vi "Diagnostic.vi"() -> ()   [LabVIEW 2018]
uses:
  Type/_GUI Method.ctl
  Type/_Lens Property.ctl
  Type/_Mass Range Property.ctl
  Type/_Mass Range Parameters.ctl
  Type/_RT Res Type.ctl
  Type/_Run Mode.ctl
  Type/_Run State.ctl
  Type/_File Type.ctl
  Type/_RT Command.ctl
  Type/_Data Operation.ctl
  Type/_Run Module.ctl
  Configuration/_Global Configuration.vi
  <vilib>/Utility/config.llb/Read Key (Path).vi
  <vilib>/Utility/config.llb/Read Key (String).vi
  <vilib>/printing/ReportDocExtensions.llb/Append Front Panel Image to Report (path).vi
  <vilib>/Utility/config.llb/Write Key (Path).vi
  <vilib>/Utility/config.llb/Write Key (String).vi
  <vilib>/Utility/miscctls.llb/LVRectTypeDef.ctl
  <vilib>/Utility/NIReport.llb/NI_report.lvclass
  <vilib>/Utility/NIReport.llb/NI_ReportGenerationCore.lvlib
  <vilib>/Utility/config.llb/NI_LVConfig.lvlib
panel:
  out "Error Out":errorcluster
  in  "Run Mode":T1
  in  "Q2DC EN":bool
  in  "Count1":dbl=400.0 caption="Lens Value" format="%#.3f"
  in  "Count2":dbl=400.0 caption="High Value" format="%#.3f"
  in  "Time1":dbl=1.0 caption="Low Dwell (ms)" format="%#.3f"
  in  "Time2":dbl=1.0 caption="High Dwell (ms)" format="%#.3f"
  in  "Scans":i32=1
  in  "Step Size":dbl=-1.0 format="%#.3f"
  in  "Scan Type":u8(ring) items=["Single", "Dual", "Ramp"]
  in  "Unit":bool
  in  "Q1DC EN":bool
  in  "Q1 POL":bool
  in  "Q2 POL":bool
  out "DAC Value":i32=98187
  in  "Lens Table":i32(listbox)
  in  "Swtich Polarity":bool
  in  "Run":bool
  out "Dual Run":bool
  out "Spectrum":cluster{"Mass":dbl[], "Data in cps":dbl[]}[](graph)=[{"Mass"=[664.0], "Data in cps"=[]}, {"Mass"=[800.0], "Data in cps"=[]}, {"Mass"=[700.0], "Data in cps"=[]}]
  in  "Cancel":bool
  in  "NewMethod":bool
  in  "Method Path":path
  in  "Method":T2={"Lenses"=[{"Scan Type"=0, "Scans"=1, "Time 1"=1.0, "Time 2"=1.0, "Value 1"=400.0, "Value 2"=400.0, "Step Size"=-1.0}, {"Scan Type"=0, "Scans"=1, "Time 1"=1.0, "Time 2"=1.0, "Value 1"=150.0, "Value 2"=150.0, "Step Size"=1.0}, {"Scan Type"=0, "Scans"=1, "Time 1"=1.0, "Time 2"=1.0, "Value 1"=32000.0, "Value 2"=32000.0, "Step Size"=1.0}, {"Scan Type"=0, "Scans"=1, "Time 1"=1.0, "Time 2"=1.0, "Value 1"=400.0, "Value 2"=400.0, "Step Size"=1.0}, {"Scan Type"=0, "Scans"=1, "Time 1"=1.0, "Time 2"=1.0, "Value 1"=150.0, "Value 2"=150.0, "Step Size"=1.0}, {"Scan Type"=0, "Scans"=1, "Time 1"=1.0, "Time 2"=1.0, "Value 1"=64000.0, "Value 2"=64000.0, "Step Size"=1.0}, {"Scan Type"=0, "Scans"=1, "Time 1"=1.0, "Time 2"=1.0, "Value 1"=420.0, "Value 2"=420.0, "Step Size"=1.0}, {"Scan Type"=0, "Scans"=1, "Time 1"=1.0, "Time 2"=1.0, "Value 1"=30.0, "Value 2"=30.0, "Step Size"=1.0}, {"Scan Type"=0, "Scans"=1, "Time 1"=1.0, "Time 2"=1.0, "Value 1"=15.0, "Value 2"=15.0, "Step Size"=1.0}, {"Scan Type"=0, "Scans"=1, "Time 1"=1.0, "Time 2"=1.0, "Value 1"=0.0, "Value 2"=0.0, "Step Size"=1.0}, {"Scan Type"=0, "Scans"=1, "Time 1"=1.0, "Time 2"=1.0, "Value 1"=0.0, "Value 2"=0.0, "Step Size"=1.0}, {"Scan Type"=0, "Scans"=1, "Time 1"=1.0, "Time 2"=1.0, "Value 1"=0.0, "Value 2"=0.0, "Step Size"=1.0}, {"Scan Type"=0, "Scans"=1, "Time 1"=1.0, "Time 2"=1.0, "Value 1"=0.0, "Value 2"=0.0, "Step Size"=1.0}, {"Scan Type"=0, "Scans"=1, "Time 1"=1.0, "Time 2"=1.0, "Value 1"=0.0, "Value 2"=0.0, "Step Size"=1.0}, {"Scan Type"=0, "Scans"=1, "Time 1"=1.0, "Time 2"=1.0, "Value 1"=-0.5, "Value 2"=-0.5, "Step Size"=1.0}, {"Scan Type"=0, "Scans"=1, "Time 1"=1.0, "Time 2"=1.0, "Value 1"=-2.0, "Value 2"=-2.0, "Step Size"=1.0}, {"Scan Type"=0, "Scans"=1, "Time 1"=1.0, "Time 2"=1.0, "Value 1"=-1.2, "Value 2"=-1.2, "Step Size"=1.0}, {"Scan Type"=0, "Scans"=1, "Time 1"=1.0, "Time 2"=1.0, "Value 1"=0.0, "Value 2"=0.0, "Step Size"=1.0}, {"Scan Type"=0, "Scans"=1, "Time 1"=1.0, "Time 2"=1.0, "Value 1"=-240.0, "Value 2"=-240.0, "Step Size"=1.0}, {"Scan Type"=0, "Scans"=1, "Time 1"=1.0, "Time 2"=1.0, "Value 1"=-50.0, "Value 2"=-50.0, "Step Size"=1.0}, {"Scan Type"=0, "Scans"=1, "Time 1"=1.0, "Time 2"=1.0, "Value 1"=-52.0, "Value 2"=-52.0, "Step Size"=1.0}, {"Scan Type"=0, "Scans"=1, "Time 1"=1.0, "Time 2"=1.0, "Value 1"=-100.0, "Value 2"=-100.0, "Step Size"=1.0}, {"Scan Type"=0, "Scans"=1, "Time 1"=1.0, "Time 2"=1.0, "Value 1"=-54.0, "Value 2"=-54.0, "Step Size"=1.0}, {"Scan Type"=0, "Scans"=1, "Time 1"=1.0, "Time 2"=1.0, "Value 1"=-400.0, "Value 2"=-400.0, "Step Size"=1.0}, {"Scan Type"=0, "Scans"=1, "Time 1"=1.0, "Time 2"=1.0, "Value 1"=30.0, "Value 2"=30.0, "Step Size"=1.0}, {"Scan Type"=0, "Scans"=1, "Time 1"=1.0, "Time 2"=1.0, "Value 1"=2000.0, "Value 2"=2000.0, "Step Size"=1.0}, {"Scan Type"=0, "Scans"=1, "Time 1"=1.0, "Time 2"=1.0, "Value 1"=-6000.0, "Value 2"=-6000.0, "Step Size"=1.0}, {"Scan Type"=0, "Scans"=1, "Time 1"=1.0, "Time 2"=1.0, "Value 1"=0.0, "Value 2"=0.0, "Step Size"=1.0}, {"Scan Type"=0, "Scans"=1, "Time 1"=1.0, "Time 2"=1.0, "Value 1"=0.0, "Value 2"=0.0, "Step Size"=1.0}, {"Scan Type"=0, "Scans"=1, "Time 1"=1.0, "Time 2"=1.0, "Value 1"=250.0, "Value 2"=250.0, "Step Size"=1.0}, {"Scan Type"=0, "Scans"=1, "Time 1"=1.0, "Time 2"=1.0, "Value 1"=-250.0, "Value 2"=-250.0, "Step Size"=1.0}, {"Scan Type"=0, "Scans"=1, "Time 1"=1.0, "Time 2"=1.0, "Value 1"=250.0, "Value 2"=250.0, "Step Size"=1.0}, {"Scan Type"=0, "Scans"=1, "Time 1"=1.0, "Time 2"=1.0, "Value 1"=-250.0, "Value 2"=-250.0, "Step Size"=1.0}, {"Scan Type"=0, "Scans"=1, "Time 1"=1.0, "Time 2"=1.0, "Value 1"=500.0, "Value 2"=500.0, "Step Size"=1.0}, {"Scan Type"=0, "Scans"=1, "Time 1"=1.0, "Time 2"=1.0, "Value 1"=-500.0, "Value 2"=-500.0, "Step Size"=1.0}, {"Scan Type"=0, "Scans"=1, "Time 1"=1.0, "Time 2"=1.0, "Value 1"=0.55, "Value 2"=0.55, "Step Size"=1.0}, {"Scan Type"=0, "Scans"=1, "Time 1"=1.0, "Time 2"=1.0, "Value 1"=0.0, "Value 2"=0.0, "Step Size"=1.0}, {"Scan Type"=0, "Scans"=1, "Time 1"=1.0, "Time 2"=1.0, "Value 1"=100.0, "Value 2"=100.0, "Step Size"=1.0}, {"Scan Type"=0, "Scans"=1, "Time 1"=1.0, "Time 2"=1.0, "Value 1"=0.0, "Value 2"=0.0, "Step Size"=1.0}, {"Scan Type"=0, "Scans"=1, "Time 1"=1.0, "Time 2"=1.0, "Value 1"=5.0, "Value 2"=5.0, "Step Size"=1.0}, {"Scan Type"=0, "Scans"=1, "Time 1"=1.0, "Time 2"=1.0, "Value 1"=0.0, "Value 2"=0.0, "Step Size"=1.0}, {"Scan Type"=0, "Scans"=1, "Time 1"=1.0, "Time 2"=1.0, "Value 1"=0.0, "Value 2"=0.0, "Step Size"=1.0}, {"Scan Type"=0, "Scans"=1, "Time 1"=1.0, "Time 2"=1.0, "Value 1"=100.0, "Value 2"=100.0, "Step Size"=1.0}, {"Scan Type"=0, "Scans"=1, "Time 1"=1.0, "Time 2"=1.0, "Value 1"=0.0, "Value 2"=0.0, "Step Size"=1.0}, {"Scan Type"=0, "Scans"=1, "Time 1"=1.0, "Time 2"=1.0, "Value 1"=5.0, "Value 2"=5.0, "Step Size"=1.0}, {"Scan Type"=0, "Scans"=1, "Time 1"=1.0, "Time 2"=1.0, "Value 1"=5000.0, "Value 2"=5000.0, "Step Size"=1.0}, {"Scan Type"=0, "Scans"=1, "Time 1"=1.0, "Time 2"=1.0, "Value 1"=0.0, "Value 2"=0.0, "Step Size"=1.0}, {"Scan Type"=0, "Scans"=1, "Time 1"=1.0, "Time 2"=1.0, "Value 1"=100.0, "Value 2"=100.0, "Step Size"=1.0}, {"Scan Type"=0, "Scans"=1, "Time 1"=1.0, "Time 2"=1.0, "Value 1"=0.0, "Value 2"=0.0, "Step Size"=1.0}, {"Scan Type"=0, "Scans"=1, "Time 1"=1.0, "Time 2"=1.0, "Value 1"=5.0, "Value 2"=5.0, "Step Size"=1.0}, {"Scan Type"=0, "Scans"=1, "Time 1"=1.0, "Time 2"=1.0, "Value 1"=1000.0, "Value 2"=1000.0, "Step Size"=1.0}, {"Scan Type"=0, "Scans"=1, "Time 1"=1.0, "Time 2"=1.0, "Value 1"=1.0, "Value 2"=1.0, "Step Size"=1.0}], "Mass Ranges"=[], "Acquire"=FALSE, "MCA"=FALSE, "Q1DC EN"=FALSE, "Q1 POL"=FALSE, "Q3 POL"=FALSE, "Q1 RF  EN"=FALSE, "Averaging"=FALSE, "Log Scale"=FALSE, "CPS"=FALSE, "Unit"=FALSE, "Data Path"=path "", "Run Mode"=enum."MRM (Q1/Q2)", "Fixed Mass (amu)"=0.0, "Q3DC EN"=FALSE, "Q3 RF  EN"=FALSE, "Negative"=FALSE} {"Mass Ranges"."Res" items=["High/High", "Medium/Medium", "Low/Low", "High/Medium", "High/Low", "Medium/High", "Medium/Low", "Low/High", "Low/Medium"]}
  out "Run Time":i32 caption="Run Time (ms)"
  in  "Log Scale":bool
  in  "Scan#":u32=1 caption="Current Scan #"
  in  "CPS":bool
  in  "Averaging":bool
  in  "MCA":bool
  in  "Acquire":bool
  in  "BloUpdate":bool
  out "Data File:":path=path "C:/Users/Min/Projects/Sniffer"
  # "Selected Lens Property"
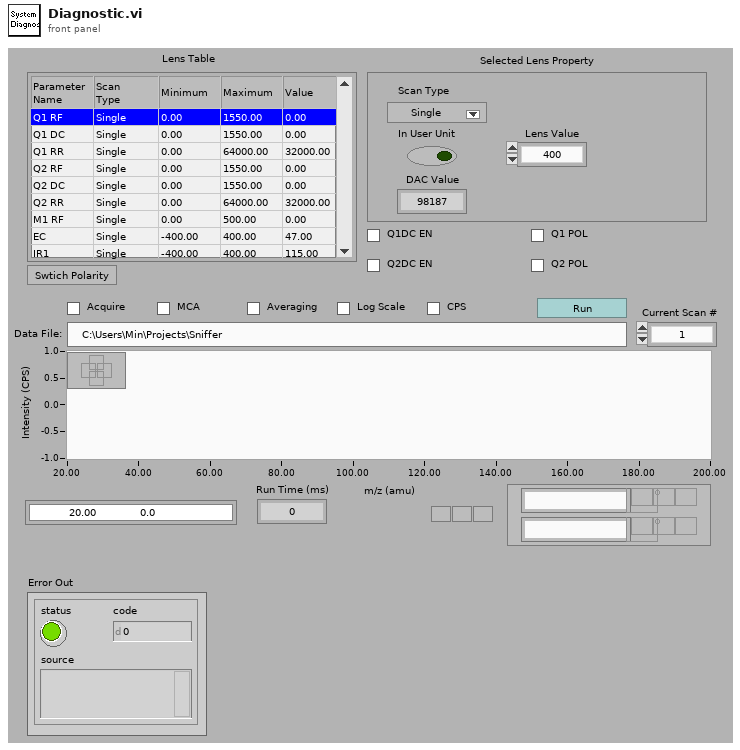
[diagram p1: front panel]
types:
  T1 = typedef "_Run Mode.ctl" = enum16{"MRM (Q1/Q2)", "Q1 Scan", "Q1 SRM", "Q2 Scan", "Q2 SRM", "Product Scan", "Precursor Scan", "Neutral Loss", "Neutral Gain"}
  T2 = typedef "_GUI Method.ctl" = cluster{"Lenses":T3[], "Mass Ranges":T4[], "Acquire":bool, "MCA":bool, "Q1DC EN":bool, "Q1 POL":bool, "Q3 POL":bool, "Q1 RF  EN":bool, "Averaging":bool, "Log Scale":bool, "CPS":bool, "Unit":bool, "Data Path":path, "Run Mode":T1, "Fixed Mass (amu)":dbl, "Q3DC EN":bool, "Q3 RF  EN":bool, "Negative":bool}
  T3 = typedef "_Lens Property.ctl" = cluster{"Scan Type":u8, "Scans":i32, "Time 1":dbl, "Time 2":dbl, "Value 1":dbl, "Value 2":dbl, "Step Size":dbl}
  T4 = typedef "_Mass Range Property.ctl" = cluster{"Start":dbl, "Stop":dbl, "Step Size":dbl, "Steps":i32, "Dwell":dbl, "Parameters":T5[], "Res":T6}
  T5 = typedef "_Mass Range Parameters.ctl" = cluster{"Name":string, "Ch#":u8, "StartV":dbl, "StopV":dbl, "StepV":dbl, "Index":u8}
  T6 = typedef "_RT Res Type.ctl" = u16
  T7 = typedef "_Run State.ctl" = enum16{"Init", "Update", "Start", "End", "Error"}
  T8 = typedef "_RT Instrument 2.ctl" = cluster{"Table":T9[], "Instrument":string[]}
  T9 = typedef "_RT Configuration 2.ctl" = cluster{"Name":string, "Ch#":u8, "Min":dbl, "Max":dbl, "Def+":dbl, "Def-":dbl, "Offset":dbl, "Slope":dbl, "Type":u8, "Description":string, "SettleT":dbl}
  T10 = typedef "_File Type.ctl" = enum16{"Configuration", "Old Configuration", "Calibration", "Resolution", "Diagnostic Method", "Old Method", "Acq Method", "Samp List"}
  T11 = typedef "LVRectTypeDef.ctl" = cluster{"Left":i16, "Top":i16, "Right":i16, "Bottom":i16}
  T12 = enum16{"Standard Report", "HTML", "Word", "Excel"}
  T13 = typedef "_RT Command.ctl" = enum16{"xml Start Run", "xml Start Actual Run", "xml Stop Run", "xml Runtime Update", "xml Get Status", "xml Get Table", "xml Set Table", "xml Get Configuration", "xml System Status", "xml Set LC Input Logic", "xml Get Data", "xml Get Info", "Start", "StartActualRun", "Stop", "Runtime Update", "Get Data", "Get Info", "Get Status", "Get Param", "Get Config", "Get Table", "Read ADC", "Set Oscillator", "Update Config", "Update Table", "Set All Pol", "Set Pol and DC", "Set Max Mass", "Toggle RP", "Toggle EL", "Set PIC", "Initialize Turbo", "Send Turbo Comm", "Close Turbo", "P1", "P2", "P3", "Send Serial", "Set LC Out", "Get LC In", "Read VAC", "Test Table", "Toggle Power", "Get Startup", "Set Startup", "Get ADC Table", "Set ADC Table", "Get Brief Status", "Get Detail Status", "Auxiliary Update", "Set CC Logics", "Set CC Input Logics", "Ignore Error", "invalid"}
  T14 = typedef "_Data Operation.ctl" = enum8{"Initialize", "Get Data", "Set Data", "Close"}
  T15 = enum32{"Bad", "Idle", "Run top level", "Running"}
  T16 = typedef "NI_LVConfig.lvlib/Config Data RefNum.ctl" = refnum<k1>
  T17 = cluster{"Method":T2, "Update":bool, "Running":bool, "Method Path":path}
  T18 = typedef "_Current Data.ctl" = cluster{"Scan#":i32, "Run Time (mS)":i32, "TIC X":dbl[], "TIC Y":dbl[][], "MassRange":cluster{"X Title":string, "X":dbl[], "Y":i32[]}[], "Fixed Mass (amu)":dbl, "Method":T19}
  T19 = typedef "_XML Expt.ctl" = cluster{"StartT(mS)":i32, "#Cycles":i32, "PauseT(uS)":i32, "ScanType":i32, "Polarity":u8, "FixedMass":dbl, "DelayT(mS)":i32, "Active Ch":T20[], "Mass Range":T4[]}
  T20 = typedef "_XML Lens.ctl" = cluster{"Value":dbl, "ChID":u8}
  T21 = cluster{"Scan Type":u8, "Unit":bool, "Count1":dbl, "Count2":dbl, "Time1":dbl, "Time2":dbl, "Scans":i32, "Step Size":dbl, "Lens Table":i32}
  T22 = cluster{"Scan Type":u8, "Unit":bool, "Count1":dbl, "Count2":dbl, "Time1":dbl, "Time2":dbl, "Scans":i32, "Step Size":dbl, "Start DAC":i32, "Ramp Time (ms)":i32}
  T23 = cluster{bool, "Value 1":dbl, "Value 2":dbl, "Step Size":dbl}
  T24 = typedef "_Run Module.ctl" = u16
  T25 = cluster{"NewVal":bool, "Count1":dbl, "Count2":dbl, "Step Size":dbl}
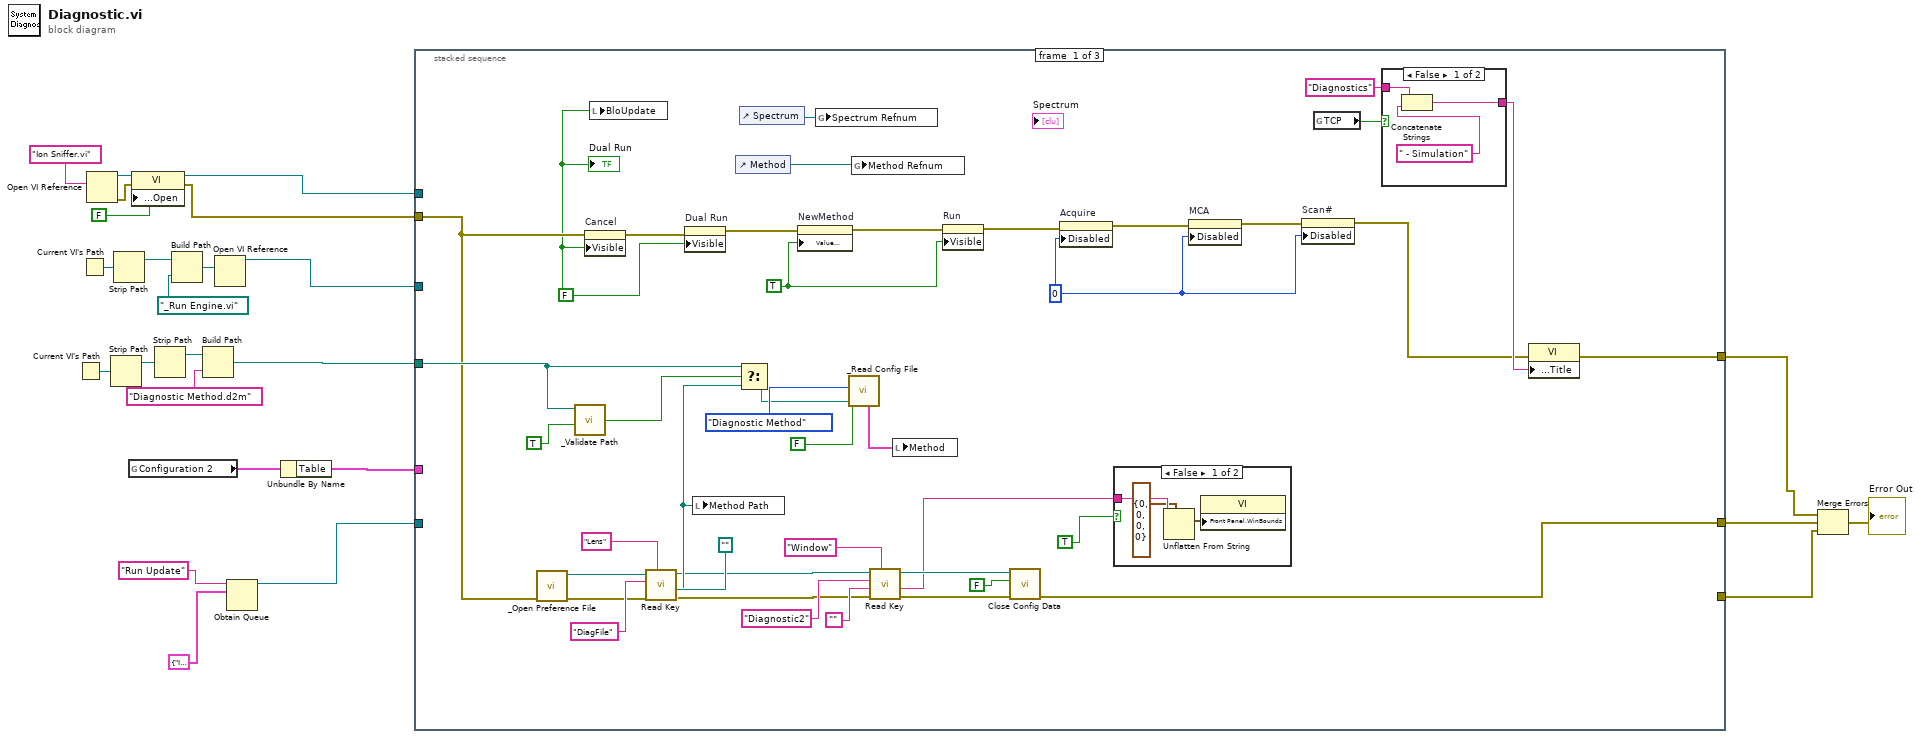
[diagram p0: block diagram]
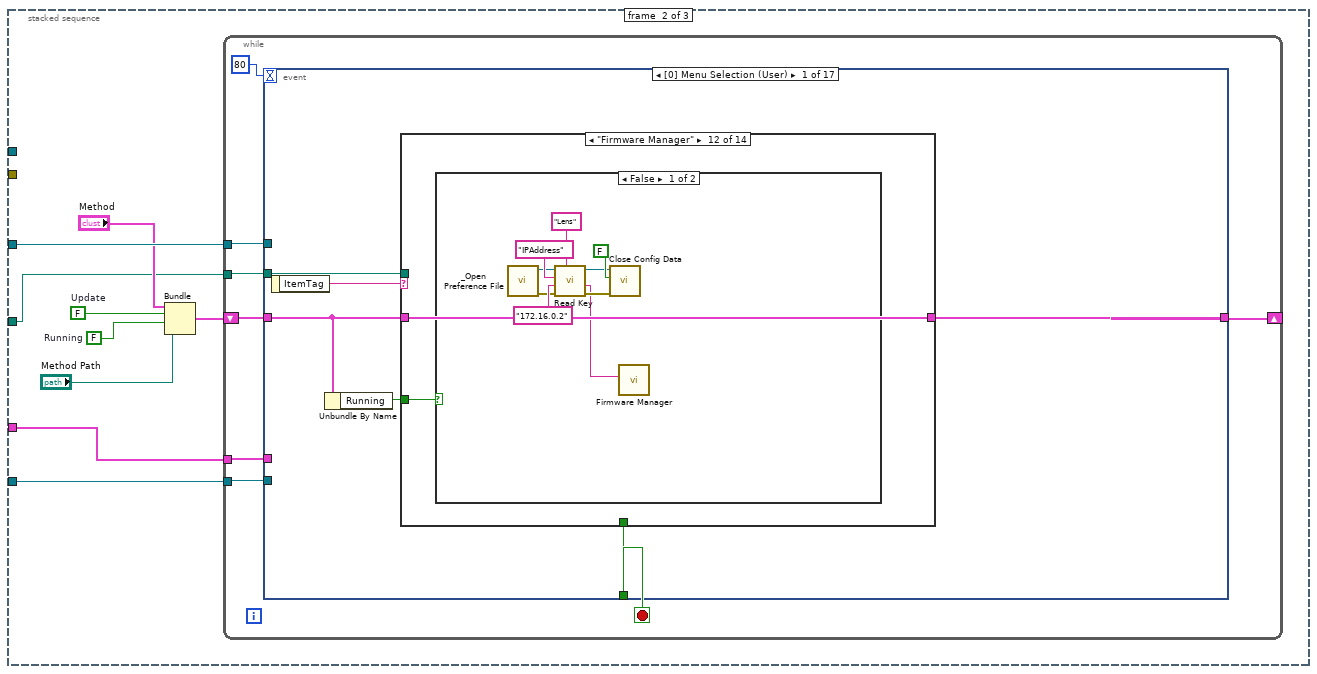
[diagram p4: hidden frame]
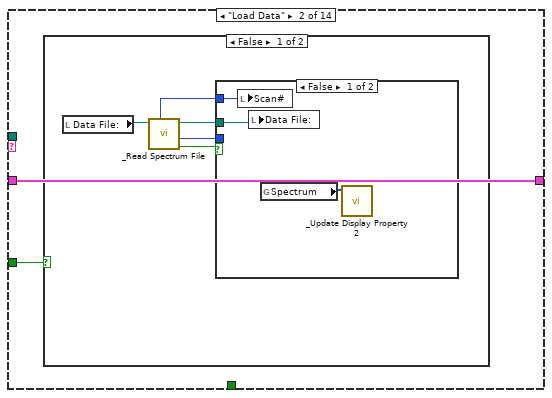
[diagram p6: hidden frame]
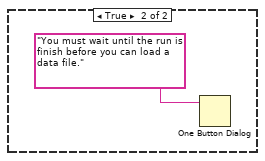
[diagram p8: hidden frame]
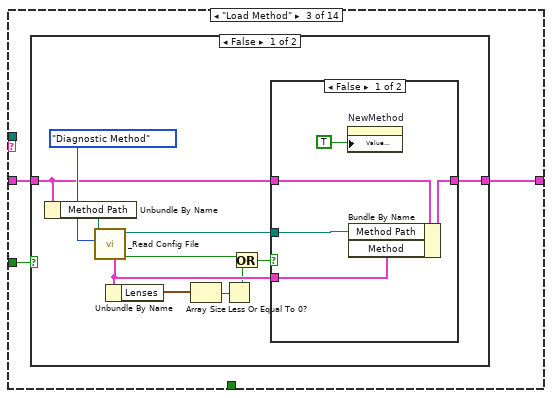
[diagram p9: hidden frame]
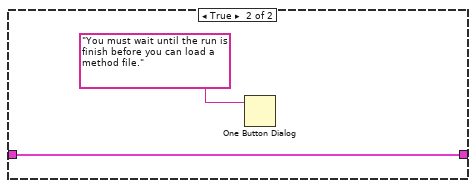
[diagram p11: hidden frame]
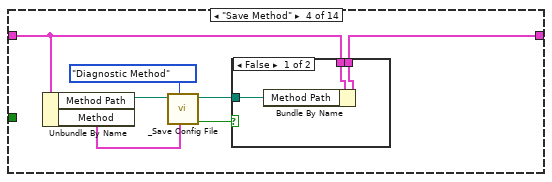
[diagram p12: hidden frame]
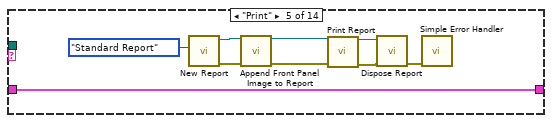
[diagram p14: hidden frame]
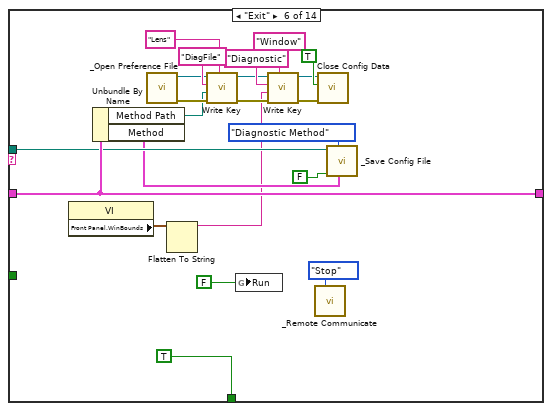
[diagram p15: hidden frame]
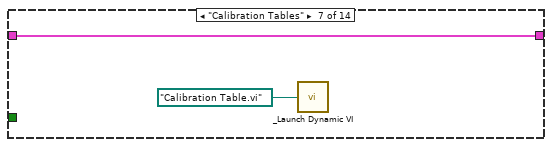
[diagram p16: hidden frame]
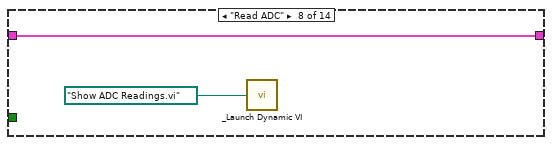
[diagram p17: hidden frame]
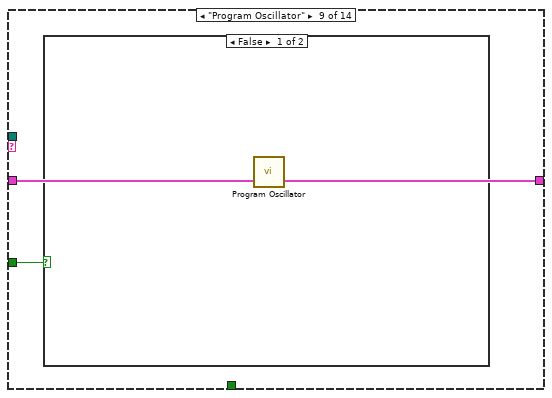
[diagram p18: hidden frame]
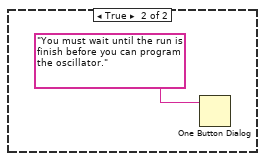
[diagram p19: hidden frame]
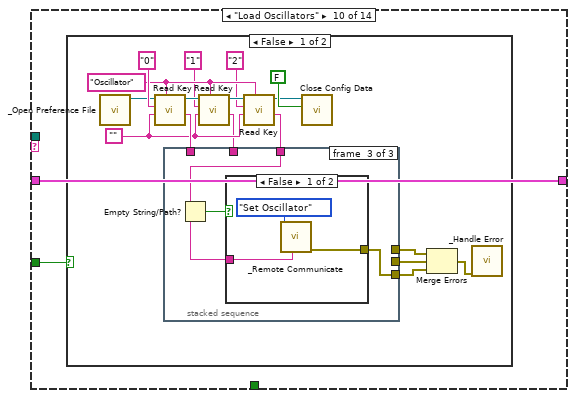
[diagram p20: hidden frame]
diagram:
  n1 = Current VI's Path() -> (path=w12:path)
  n2 = Current VI's Path() -> (path=w22:path)
  n3 = Open VI Reference(vi path="Ion Sniffer.vi") -> (vi reference=w9:refnum<vi>, error out=w8:errorcluster)  [unwired: 1 in, 4 out]
  n4 = Strip Path(path=w12) -> (stripped path=w13:path)  [unwired: 1 out]
  n5 = Strip Path(path=w22) -> (stripped path=w18:path)  [unwired: 1 out]
  n6 = global read "_Global Configuration.vi" "Configuration 2"() -> (w17:T8)
  n7 = property class="VI"(reference=w9, error in=w8, "Front Panel Window:Open"=FALSE) -> (reference out=w6:refnum<vi>, error out=w5:errorcluster)
  n8 = Strip Path(path=w13) -> (stripped path=w14:path)  [unwired: 1 out]
  n9 = Build Path(base path=w18, name or relative path=path "_Run Engine.vi") -> (appended path=w20:path)
  n10 = Build Path(base path=w14, name or relative path="Diagnostic Method.d2m") -> (appended path=w11:path)
  n11 = Open VI Reference(vi path=w20) -> (vi reference=w19:refnum<vi>)  [unwired: 1 in, 5 out]
  n12 = Obtain Queue(name (unnamed)="Run Update", element data type=cluster{T7, dbl, "error out":errorcluster} {enum."Init", 0.0, "error out"={"status"=FALSE, "code"=0, "source"=""}}) -> (queue out=w23:refnum<queue>)  [unwired: 3 in, 2 out]
  n13 = Unbundle By Name(w17) -> ("Table"=w16:T9[])
  n14 = stacked-sequence {
    tunnel: w23 -> [_ w82 w647]
    tunnel: w19 -> [_ w81 w646]
    tunnel: w16 -> [_ w75 _]
    tunnel: w11 -> [w39 w74 _]
    tunnel: w6 -> [_ _ w642]
    tunnel: w5 -> [w36 _ w641]
    tunnel: [_ _ w638] -> w2
    tunnel: [w27 _ _] -> w3
    tunnel: [w26 _ _] -> w1
    frame #0 {
      w43 = TRUE ("Visible")
      w63 = u8 0 ("Disabled")
      w32 = FALSE ("Unit")
      n15 = call "_Open Preference File.vi"("error In"=w36) -> ("error"=w59:errorcluster, "refnum"=w60:T16)  [unwired: 2 in, 3 out]
      n16 = call "_Validate Path.vi"("Check Exist (F)"=TRUE, "path"=w39) -> ("Valid"=w40:bool)  [unwired: 2 in]
      n17 = property on="Cancel" class="Bool"(error in=w36, "Visible"=w32) -> (error out=w35:errorcluster)  [unwired: 1 in, 1 out]
      n18 = local write "BloUpdate"(w32) -> ()
      n19 = call-poly <vilib>:"Read Key.vi"("section"="Lens", "error in (no error)"=w59, "default value"=path "", "key"="DiagFile", "refnum"=w60) -> ("error out"=w47:errorcluster, "value"=w53:path, "refnum out"=w48:T16)  [unwired: 4 out]
      n20 = property on="Dual Run" class="Bool (strict)"(error in=w35, "Visible"=w32) -> (error out=w34:errorcluster)  [unwired: 1 in, 1 out]
      n21 = local write "Method Path"(w53) -> ()
      n22 = control-ref of="Method"() -> (w41:refnum<vi>)
      n23 = Select(t=w39, s=w40, f=w53) -> (s? t:f=w52:path)
      n24 = control-ref of="Spectrum"() -> (w42:refnum<vi>)
      n25 = property on="NewMethod" class="Bool (strict)"(error in=w34, "Value (Signaling)"=w43) -> (error out=w33:errorcluster)  [unwired: 1 in, 1 out]
      n26 = global write "_Global Configuration.vi" "Spectrum Refnum"(w42) -> ()
      n27 = call "_Read Config File.vi"("advisory dialog? (display:T)"=FALSE, "File Type (config)"=_File_Type."Diagnostic Method", "start path  (Not A Path)"=w52) -> ("GUI Method"=w55:T2)  [unwired: 8 out]
      n28 = global write "_Global Configuration.vi" "Method Refnum"(w41) -> ()
      n29 = call-poly <vilib>:"Read Key.vi"("section"="Window", "error in (no error)"=w47, "default value"="", "key"="Diagnostic2" ("section"), "refnum"=w48) -> ("error out"=w45:errorcluster, "value"=w44:string, "refnum out"=w46:T16)  [unwired: 1 in, 3 out]
      n30 = local write "Method"(w55) -> ()
      n31 = property on="Run" class="Bool"(error in=w33, "Visible"=w43) -> (error out=w31:errorcluster)  [unwired: 1 in, 1 out]
      n32 = call <vilib>:"Close Config Data.vi"("error in (no error)"=w45, "write file if changed (T)"=FALSE ("write configuration file? (F)"), "refnum"=w46) -> ("error out"=w26:errorcluster)  [unwired: 8 out]
      n33 = property on="Acquire" class="Bool (strict)"(error in=w31, "Disabled"=w63) -> (error out=w30:errorcluster)  [unwired: 1 in, 1 out]
      n34 = case shown="False" TRUE {
        tunnel: w44 -> [w69 _]
        frame False {
          n35 = Unflatten From String(type=T11 {"Left"=0, "Top"=0, "Right"=0, "Bottom"=0} ("Front Panel Window:Window Bounds"), binary string=w69) -> (value=w67:T11)  [unwired: 1 in, 4 out]
          n36 = property class="VI"("Front Panel.WinBounds"=w67) -> ()  [unwired: 2 in, 2 out]
        }
        frame True {
        }
      }
      n37 = property on="MCA" class="Bool (strict)"(error in=w30, "Disabled"=w63) -> (error out=w29:errorcluster)  [unwired: 1 in, 1 out]
      n38 = property on="Scan#" class="DigNum (strict)"(error in=w29, "Disabled"=w63) -> (error out=w28:errorcluster)  [unwired: 1 in, 1 out]
      n39 = global read "_Global Configuration.vi" "TCP"() -> (w64:bool)
      n40 = case shown="False" w64 {
        tunnel: "Diagnostics" ("string") -> [w72 w73]
        tunnel: [w70 w73] -> w65
        frame False {
          n41 = Concatenate Strings(w72, " - Simulation" ("string")) -> (w70:string)
        }
        frame True {
        }
      }
      n42 = property class="VI"(error in=w28, "Front Panel Window:Title"=w65) -> (error out=w27:errorcluster)  [unwired: 1 in, 1 out]
      "Dual Run" <- w32
    }
    frame #1 {
      w78 = FALSE  # Running
      w79 = FALSE  # Update
      n43 = Bundle("Method"="Method", "Update"=w79, "Running"=w78, "Method Path"="Method Path") -> (w77:T17)  [unwired: 1 out]
      n44 = while {
        shift-right: [w87] -> _
        shift-left: w77 -> [w89]
        tunnel: w82 -> [w86]
        tunnel: w81 -> [w85]
        tunnel: w75 -> [w84]
        tunnel: w74 -> [w83]
        stop <- w90 stop-if-true
        n45 = event shown="[0] Menu Selection (User)" {
          selector: _ -> [_ _ _ _ _ _ _ _ _ _ _ _ _ _ _ _ _]
          dyn-events: _ -> [_ _ _ _ _ _ _ _ _ _ _ _ _ _ _ _ _]
          timeout: 80 -> [_ _ _ _ _ _ _ _ _ _ _ _ _ _ _ _ _]
          tunnel: [w94 w273 _ _ _ _ _ _ _ _ _ _ _ _ _ _ _] -> w90
          tunnel: w89 -> [w93 w265 w276 w352 w396 w426 w461 w483 w496 w550 w566 w586 w600 w602 w619 w623 w637]
          tunnel: [w95 w265 w278 w352 w395 w423 w460 w483 w495 w551 w579 w585 w596 w602 w618 w622 w635] -> w87
          tunnel: w86 -> [_ _ w277 _ _ w427 _ _ _ _ _ _ _ _ _ _ _]
          tunnel: w85 -> [_ _ _ _ _ w428 w459 _ _ _ _ _ _ _ _ _ _]
          tunnel: w84 -> [_ _ _ w349 _ _ _ _ w499 _ _ _ _ _ _ w627 _]
          tunnel: w83 -> [w91 w262 _ _ _ _ _ _ _ _ _ _ _ _ _ _ _]
          event Menu Selection (User) {
            n46 = event-data() -> ("ItemTag"=w96:string)  [unwired: 1 out]
            n47 = Unbundle By Name(w93) -> ("Running"=w92:bool)
            n48 = case shown="\"Firmware Manager\"" w96 {
              tunnel: w92 -> [_ w99 w111 _ _ _ _ _ w178 w181 w225 w239 _ _]
              tunnel: w93 -> [w97 w98 w110 w132 w144 w166 w173 w175 w177 w180 w224 w238 w250 w251]
              tunnel: [w97 w98 w109 w131 w144 w166 w173 w175 w177 w180 w224 w238 w250 w251] -> w95
              tunnel: [_ _ _ _ _ TRUE _ _ _ _ _ _ _ _] -> w94
              tunnel: w91 -> [_ _ _ _ _ w160 _ _ _ _ _ _ _ _]
              frame Default {
              }
              frame "Load Data" {
                n49 = case shown="False" w99 {
                  frame False {
                    n50 = local read "Data File:"() -> (w102:path)
                    n51 = call "_Read Spectrum File.vi"("start path  (Not A Path)"=w102) -> ("error"=w104:bool, "TIC"=w103:u32, "new file path"=w101:path, "Scan# out"=w100:u32)  [unwired: 2 in, 3 out]
                    n52 = case shown="False" w104 {
                      tunnel: w103 -> [_ _]
                      tunnel: w101 -> [w107 _]
                      tunnel: w100 -> [w106 _]
                      frame False {
                        n53 = local write "Scan#"(w106) -> ()
                        n54 = local write "Data File:"(w107) -> ()
                        n55 = global read "_Global Configuration.vi" "Spectrum"() -> (w105:i32[])
                        n56 = call "_Update Display Property 2.vi"("Spectrum in"=w105) -> ()  [unwired: 7 out]
                      }
                      frame True {
                      }
                    }
                  }
                  frame True {
                    n57 = One Button Dialog(message="You must wait until the run is finish before you can load a data file.") -> ()  [unwired: 2 out]
                  }
                }
              }
              frame "Load Method" {
                n58 = case shown="False" w111 {
                  tunnel: w110 -> [w120 w129]
                  tunnel: [w112 w129] -> w109
                  frame False {
                    n59 = Unbundle By Name(w120) -> ("Method Path"=w122:path)
                    n60 = call "_Read Config File.vi"("File Type (config)"=_File_Type."Diagnostic Method", "start path  (Not A Path)"=w122) -> ("error"=w115:bool, "new file path"=w119:path, "GUI Method"=w118:T2)  [unwired: 1 in, 6 out]
                    n61 = Unbundle By Name(w118) -> ("Lenses"=w117:T3[])
                    n62 = Array Size(array=w117) -> (size(s)=w116:i32)
                    n63 = Less Or Equal To 0?(x=w116) -> (x <= 0?=w114:bool)
                    n64 = Or(x=w115, y=w114) -> (x .or. y?=w113:bool)
                    n65 = case shown="False" w113 {
                      tunnel: w120 -> [w127 w128]
                      tunnel: w118 -> [w124 _]
                      tunnel: w119 -> [w125 _]
                      tunnel: [w126 w128] -> w112
                      frame False {
                        n66 = property on="NewMethod" class="Bool (strict)"("Value (Signaling)"=TRUE) -> ()  [unwired: 2 in, 2 out]
                        n67 = Bundle By Name(cluster=w127, "Method Path"=w125, "Method"=w124) -> (w126:T17)
                      }
                      frame True {
                      }
                    }
                  }
                  frame True {
                    n68 = One Button Dialog(message="You must wait until the run is finish before you can load a method file.") -> ()  [unwired: 2 out]
                  }
                }
              }
              frame "Save Method" {
                n69 = Unbundle By Name(w132) -> ("Method Path"=w135:path, "Method"=w133:T2)
                n70 = call "_Save Config File.vi"("GUI Method"=w133, "File Type (config)"=_File_Type."Diagnostic Method", "start path  (Not A Path)"=w135) -> ("error"=w136:bool, "new file path"=w137:path)  [unwired: 5 in, 2 out]
                n71 = case shown="False" w136 {
                  tunnel: w137 -> [w139 _]
                  tunnel: w132 -> [w140 w141]
                  tunnel: [w138 w141] -> w131
                  frame False {
                    n72 = Bundle By Name(cluster=w140, "Method Path"=w139) -> (w138:T17)
                  }
                  frame True {
                  }
                }
              }
              frame "Print" {
                n73 = call <vilib>:"New Report.vi"("report type"=T12."Standard Report") -> ("report out"=w148:refnum<class "NI_report.lvclass">, "error out"=w147:errorcluster)  [unwired: 5 in, 8 out]
                n74 = call-poly <vilib>:"Append Front Panel Image to Report.vi"("report in"=w148, "error in (no error)"=w147) -> ("report out"=w146:refnum<class "NI_report.lvclass">, "error out"=w145:errorcluster)  [unwired: 6 in, 6 out]
                n75 = call-dynamic "Print Report.vi"("report in"=w146, "error in (no error)"=w145) -> ("report out"=w150:refnum<class "NI_report.lvclass">, "error out"=w149:errorcluster)  [unwired: 2 in, 10 out]
                n76 = call-dynamic "Dispose Report.vi"("report in"=w150, "error in (no error)"=w149) -> ("error out"=w143:errorcluster)  [unwired: 3 in, 10 out]
                n77 = call <vilib>:"Simple Error Handler.vi"("error in (no error)"=w143) -> ()  [unwired: 1 in, 8 out]
              }
              frame "Exit" {
                n78 = property class="VI"() -> ("Front Panel.WinBounds"=w152:T11)  [unwired: 2 in, 2 out]
                n79 = Unbundle By Name(w166) -> ("Method Path"=w167:path, "Method"=w159:T2)
                n80 = call "_Open Preference File.vi"() -> ("error"=w168:errorcluster, "refnum"=w169:T16)  [unwired: 3 in, 3 out]
                n81 = Flatten To String(anything=w152) -> (data string=w151:string)  [unwired: 1 in, 4 out]
                n82 = call-poly <vilib>:"Write Key.vi"("section"="Lens", "error in (no error)"=w168, "value"=w167, "key"="DiagFile", "refnum"=w169) -> ("error out"=w154:errorcluster, "refnum out"=w156:T16)  [unwired: 5 out]
                n83 = global write "_Global Configuration.vi" "Run"(FALSE ("Update")) -> ()
                n84 = call-poly <vilib>:"Write Key.vi"("section"="Window", "error in (no error)"=w154, "value"=w151, "key"="Diagnostic" ("section"), "refnum"=w156) -> ("error out"=w153:errorcluster, "refnum out"=w155:T16)  [unwired: 1 in, 4 out]
                n85 = call "_Remote Communicate.vi"("Command"=_RT_Command."Stop") -> ()  [unwired: 5 in, 4 out]
                n86 = call <vilib>:"Close Config Data.vi"("error in (no error)"=w153, "write file if changed (T)"=TRUE ("write configuration file? (F)"), "refnum"=w155) -> ()  [unwired: 9 out]
                n87 = call "_Save Config File.vi"("GUI Method"=w159, "File Type (config)"=_File_Type."Diagnostic Method", "advisory dialog? (display:T)"=FALSE, "start path  (Not A Path)"=w160) -> ()  [unwired: 4 in, 4 out]
              }
              frame "Calibration Tables" {
                n88 = call "_Launch Dynamic VI.vi"("VI Name"=path "Calibration Table.vi" ("name or relative path")) -> ()  [unwired: 3 in, 1 out]
              }
              frame "Read ADC" {
                n89 = call "_Launch Dynamic VI.vi"("VI Name"=path "Show ADC Readings.vi" ("name or relative path")) -> ()  [unwired: 3 in, 1 out]
              }
              frame "Program Oscillator" {
                n90 = case shown="False" w178 {
                  frame False {
                    n91 = call "Program Oscillator.vi"() -> ()  [unwired: 1 out]
                  }
                  frame True {
                    n92 = One Button Dialog(message="You must wait until the run is finish before you can program the oscillator.") -> ()  [unwired: 2 out]
                  }
                }
              }
              frame "Load Oscillators" {
                n93 = case shown="False" w181 {
                  frame False {
                    w188 = ""
                    w194 = "Oscillator" ("section")
                    n94 = call "_Open Preference File.vi"() -> ("refnum"=w197:T16)  [unwired: 3 in, 4 out]
                    n95 = call-poly <vilib>:"Read Key.vi"("section"=w194, "default value"=w188, "key"="0" ("section"), "refnum"=w197) -> ("value"=w189:string, "refnum out"=w196:T16)  [unwired: 2 in, 4 out]
                    n96 = call-poly <vilib>:"Read Key.vi"("section"=w194, "default value"=w188, "key"="1" ("section"), "refnum"=w196) -> ("value"=w187:string, "refnum out"=w195:T16)  [unwired: 2 in, 4 out]
                    n97 = call-poly <vilib>:"Read Key.vi"("section"=w194, "default value"=w188, "key"="2" ("section"), "refnum"=w195) -> ("value"=w186:string, "refnum out"=w190:T16)  [unwired: 2 in, 4 out]
                    n98 = stacked-sequence {
                      tunnel: w189 -> [w200 _ _]
                      tunnel: [w199 _ _] -> w185
                      tunnel: w187 -> [_ w208 _]
                      tunnel: w186 -> [_ _ w216]
                      tunnel: [_ w207 _] -> w184
                      tunnel: [_ _ w215] -> w183
                      frame #0 {
                        n99 = Empty String/Path?(string/path=w200) -> (empty?=w201:bool)
                        n100 = case shown="False" w201 {
                          tunnel: w200 -> [w203 _]
                          tunnel: [w202 w206] -> w199
                          frame False {
                            n101 = call "_Remote Communicate.vi"("String"=w203, "Command"=_RT_Command."Set Oscillator") -> ("error out"=w202:errorcluster)  [unwired: 4 in, 3 out]
                          }
                          frame True {
                            n102 = call "_Construct Error Cluster.vi"("reason"="Q1-FREQ has not been programmed.") -> ("error out"=w206:errorcluster)  [unwired: 3 in, 3 out]
                          }
                        }
                      }
                      frame #1 {
                        n103 = Empty String/Path?(string/path=w208) -> (empty?=w209:bool)
                        n104 = case shown="False" w209 {
                          tunnel: w208 -> [w211 _]
                          tunnel: [w210 w214] -> w207
                          frame False {
                            n105 = call "_Remote Communicate.vi"("String"=w211, "Command"=_RT_Command."Set Oscillator") -> ("error out"=w210:errorcluster)  [unwired: 4 in, 3 out]
                          }
                          frame True {
                            n106 = call "_Construct Error Cluster.vi"("reason"="Q3-FREQ has not been programmed.") -> ("error out"=w214:errorcluster)  [unwired: 3 in, 3 out]
                          }
                        }
                      }
                      frame #2 {
                        n107 = Empty String/Path?(string/path=w216) -> (empty?=w217:bool)
                        n108 = case shown="False" w217 {
                          tunnel: w216 -> [w219 _]
                          tunnel: [w218 w222] -> w215
                          frame False {
                            n109 = call "_Remote Communicate.vi"("String"=w219, "Command"=_RT_Command."Set Oscillator") -> ("error out"=w218:errorcluster)  [unwired: 4 in, 3 out]
                          }
                          frame True {
                            n110 = call "_Construct Error Cluster.vi"("reason"="MP1-FREQ has not been programmed.") -> ("error out"=w222:errorcluster)  [unwired: 3 in, 3 out]
                          }
                        }
                      }
                    }
                    n111 = call <vilib>:"Close Config Data.vi"("write file if changed (T)"=FALSE ("write configuration file? (T)"), "refnum"=w190) -> ()  [unwired: 1 in, 9 out]
                    n112 = Merge Errors(w185, w184, w183) -> (w182:errorcluster)
                    n113 = call "_Handle Error.vi"("error in (no error)"=w182) -> ()  [unwired: 2 in, 5 out]
                  }
                  frame True {
                    n114 = One Button Dialog(message="You must wait until the run is finish before you can load the oscillators.") -> ()  [unwired: 2 out]
                  }
                }
              }
              frame "Firmware Reboot" {
                n115 = case shown="False" w225 {
                  frame False {
                    n116 = Two Button Dialog(message="You will have to wait up to 3 min for the firmware to finish rebooting.  Proceed? ") -> (T button?=w226:bool)  [unwired: 2 out]
                    n117 = case shown="True" w226 {
                      frame False {
                      }
                      frame True {
                        n118 = call "_Open Preference File.vi"() -> ("error"=w229:errorcluster, "refnum"=w230:T16)  [unwired: 3 in, 3 out]
                        n119 = call-poly <vilib>:"Read Key.vi"("section"="Lens", "error in (no error)"=w229, "default value"="172.16.0.2", "key"="IPAddress", "refnum"=w230) -> ("error out"=w231:errorcluster, "value"=w228:string, "refnum out"=w232:T16)  [unwired: 1 in, 3 out]
                        n120 = call "_Remote Reboot.vi"("IP Address"=w228) -> ()  [unwired: 2 out]
                        n121 = call <vilib>:"Close Config Data.vi"("error in (no error)"=w231, "write file if changed (T)"=FALSE ("write configuration file? (F)"), "refnum"=w232) -> ()  [unwired: 9 out]
                      }
                    }
                  }
                  frame True {
                    n122 = One Button Dialog(message="You must wait until the run is finish before you can reboot the firware.") -> ()  [unwired: 2 out]
                  }
                }
              }
              frame "Firmware Manager" {
                n123 = case shown="False" w239 {
                  frame False {
                    n124 = call "_Open Preference File.vi"() -> ("error"=w241:errorcluster, "refnum"=w242:T16)  [unwired: 3 in, 3 out]
                    n125 = call-poly <vilib>:"Read Key.vi"("section"="Lens", "error in (no error)"=w241, "default value"="172.16.0.2", "key"="IPAddress", "refnum"=w242) -> ("error out"=w243:errorcluster, "value"=w240:string, "refnum out"=w244:T16)  [unwired: 1 in, 3 out]
                    n126 = call <vilib>:"Close Config Data.vi"("error in (no error)"=w243, "write file if changed (T)"=FALSE ("write configuration file? (F)"), "refnum"=w244) -> ()  [unwired: 9 out]
                    n127 = call "Firmware Manager.vi"("cRIO IP Address"=w240) -> ()  [unwired: 2 in, 5 out]
                  }
                  frame True {
                    n128 = One Button Dialog(message="You must wait until the run is finish before you can backup or update the firware.") -> ()  [unwired: 2 out]
                  }
                }
              }
              frame "Read FPGA Map" {
                n129 = call "Show FPGA Map.vi"() -> ()  [unwired: 12 out]
              }
              frame "About" {
                n130 = call "About Box.vi"() -> ()  [unwired: 1 out]
              }
            }
          }
          event Panel Close? {
            w273 = TRUE ("Discard?")
            n131 = event-data() -> ()  [unwired: 4 out]
            n132 = property class="VI"() -> ("Front Panel.WinBounds"=w253:T11)  [unwired: 2 in, 2 out]
            n133 = Unbundle By Name(w265) -> ("Method Path"=w264:path, "Method"=w261:T2)
            n134 = call "_Remote Communicate.vi"("Command"=_RT_Command."Stop") -> ()  [unwired: 5 in, 4 out]
            n135 = Flatten To String(anything=w253) -> (data string=w252:string)  [unwired: 1 in, 4 out]
            n136 = call "_Open Preference File.vi"() -> ("error"=w268:errorcluster, "refnum"=w269:T16)  [unwired: 3 in, 3 out]
            n137 = call-poly <vilib>:"Write Key.vi"("section"="Lens", "error in (no error)"=w268, "value"=w264, "key"="DiagFile", "refnum"=w269) -> ("error out"=w256:errorcluster, "refnum out"=w257:T16)  [unwired: 5 out]
            n138 = call-poly <vilib>:"Write Key.vi"("section"="Window", "error in (no error)"=w256, "value"=w252, "key"="Diagnostic2" ("section"), "refnum"=w257) -> ("error out"=w254:errorcluster, "refnum out"=w255:T16)  [unwired: 1 in, 4 out]
            n139 = call <vilib>:"Close Config Data.vi"("error in (no error)"=w254, "write file if changed (T)"=TRUE ("write configuration file? (F)"), "refnum"=w255) -> ()  [unwired: 9 out]
            n140 = call "_Save Config File.vi"("GUI Method"=w261, "File Type (config)"=_File_Type."Diagnostic Method", "advisory dialog? (display:T)"=FALSE, "start path  (Not A Path)"=w262) -> ()  [unwired: 4 in, 4 out]
            n141 = global write "_Global Configuration.vi" "Run"(FALSE ("Update")) -> ()
            n142 = event-data("Discard?"=w273) -> ()  [unwired: 1 in, 1 out]
          }
          event Timeout {
            n143 = event-data() -> ()  [unwired: 4 out]
            n144 = Unbundle By Name(w276) -> ("Update"=w275:bool, "Running"=w274:bool)
            n145 = case shown="False" w275 {
              tunnel: w276 -> [w280 w324]
              tunnel: [w279 w322] -> w278
              tunnel: w274 -> [w282 _]
              tunnel: w277 -> [w281 _]
              frame False {
                n146 = case shown="True" w282 {
                  tunnel: w281 -> [_ w289]
                  tunnel: w280 -> [w283 w285]
                  tunnel: [w283 w284] -> w279
                  frame False {
                  }
                  frame True {
                    n147 = Dequeue Element(queue=w289, timeout in ms (-1)=1) -> (element=w287:cluster{T7, dbl, "error out":errorcluster}, timed out?=w286:bool)  [unwired: 1 in, 2 out]
                    n148 = case shown="False" w286 {
                      tunnel: w287 -> [w295 _]
                      tunnel: w285 -> [w291 w312]
                      tunnel: [w290 w312] -> w284
                      frame False {
                        n149 = Unbundle(w295) -> (w294:T7, w292:dbl, "error out"=w293:errorcluster)
                        n150 = case shown="\"End\"" w294 {
                          tunnel: w293 -> [_ w301 w305]
                          tunnel: w292 -> [_ _ _]
                          tunnel: w291 -> [w296 w300 w304]
                          tunnel: [w296 w299 w304] -> w290
                          frame "Init", Default {
                          }
                          frame "End" {
                            w302 = u8 0 ("Disabled")
                            n151 = property on="Run" class="Bool"("Visible"=TRUE) -> ()  [unwired: 2 in, 2 out]
                            n152 = property on="Cancel" class="Bool"("Visible"=FALSE) -> ()  [unwired: 2 in, 2 out]
                            n153 = call "_Handle Error.vi"("error in (no error)"=w301) -> ()  [unwired: 2 in, 5 out]
                            n154 = property on="Acquire" class="Bool (strict)"("Disabled"=w302) -> ()  [unwired: 2 in, 2 out]
                            n155 = property on="MCA" class="Bool (strict)"("Disabled"=w302) -> ()  [unwired: 2 in, 2 out]
                            n156 = property on="Scan#" class="DigNum (strict)"("Disabled"=w302) -> ()  [unwired: 2 in, 2 out]
                            n157 = Bundle By Name(cluster=w300, "Running"=FALSE) -> (w299:T17)
                          }
                          frame "Error" {
                            n158 = call "_Handle Error.vi"("error in (no error)"=w305) -> ()  [unwired: 2 in, 5 out]
                          }
                        }
                      }
                      frame True {
                        n159 = call "_Current Data Global.vi"("Operation"=_Data_Operation."Get Data") -> ("Latest Raw Data"=w308:i32[], "CurrentData"=w307:T18[])  [unwired: 3 in, 2 out]
                        n160 = global write "_Global Configuration.vi" "Spectrum"(w308) -> ()
                        n161 = call "_Update Display Property 2.vi"("Spectrum in"=w308) -> ()  [unwired: 7 out]
                        n162 = Index Array(array=w307) -> (element=w306:T18)  [unwired: 1 in]
                        n163 = Unbundle By Name(w306) -> ("Scan#"=w310:i32, "Run Time (mS)"=w309:i32)
                        n164 = local write "Run Time"(w309) -> ()
                        n165 = local write "Scan#"(w310) -> ()
                      }
                    }
                  }
                }
              }
              frame True {
                n166 = Unbundle By Name(w324) -> ("Method.Unit"=w321:bool, "Method"=w325:T2)
                n167 = property on="BloUpdate" class="Bool (strict)"("Value (Signaling)"=TRUE) -> ()  [unwired: 2 in, 2 out]
                n168 = Bundle("Scan Type"="Scan Type", "Unit"=w321, "Count1"="Count1", "Count2"="Count2", "Time1"="Time1", "Time2"="Time2", "Scans"="Scans", "Step Size"="Step Size", "Lens Table"="Lens Table") -> (w333:T21)  [unwired: 1 out]
                n169 = call "_Validate Lens Property.vi"("Lens Property In"=w333, "Method In"=w325) -> ("Lens Table"=w327:string[][], "Lens Property Out"=w332:T22, "Method Out"=w319:T2)  [unwired: 2 in, 2 out]
                n170 = property on="Lens Table" class="MCListbox (strict)"("Item Names"=w327) -> ()  [unwired: 2 in, 2 out]
                n171 = local write "Method"(w319) -> ()
                n172 = Bundle By Name(cluster=w324, "Method"=w319, "Update"=FALSE) -> (w322:T17)
                n173 = Unbundle By Name(w332) -> ("Scan Type"=w326:u8, "Unit"=w320:bool, "Count1"=w330:dbl, "Count2"=w329:dbl, "Time1"=w313:dbl, "Time2"=w314:dbl, "Scans"=w328:i32, "Step Size"=w331:dbl, "Start DAC"=→"DAC Value":i32, "Ramp Time (ms)"=→"Run Time":i32)
                n174 = local write "Unit"(w320) -> ()
                n175 = local write "Count1"(w330) -> ()
                n176 = local write "Count2"(w329) -> ()
                n177 = local write "Time1"(w313) -> ()
                n178 = local write "Time2"(w314) -> ()
                n179 = local write "Scan Type"(w326) -> ()
                n180 = local write "Scans"(w328) -> ()
                n181 = local write "Step Size"(w331) -> ()
              }
            }
          }
          event "Lens Table": Value Change {
            n182 = event-data() -> ("NewVal"=w357:i32)  [unwired: 1 out]
            n183 = Unbundle By Name(w352) -> ("Method.Unit"=w341:bool, "Method.Lenses"=w353:T3[])
            n184 = Array Size(array=w353) -> (size(s)=w354:i32)
            n185 = Decrement(x=w354) -> (x-1=w355:i32)
            n186 = In Range and Coerce(upper limit=w355, x=w357, lower limit=0) -> (coerced(x)=w348:i32)  [unwired: 1 out]
            n187 = local write "Lens Table"(w348) -> ()
            n188 = Index Array(array=w353, index=w348) -> (element=w351:T3)
            n189 = Index Array(array=w349, index=w348) -> (element=w344:T9)
            n190 = Unbundle By Name(w351) -> ("Scan Type"=w350:u8, "Value 1"=w361:dbl, "Value 2"=w360:dbl, "Time 1"=w359:dbl, "Time 2"=w365:dbl, "Scans"=w364:i32, "Step Size"=w362:dbl)
            n191 = Unbundle By Name(w344) -> ("Ch#"=w347:u8, "Slope"=w346:dbl, "Offset"=w345:dbl)
            n192 = local write "Time1"(w359) -> ()
            n193 = local write "Time2"(w365) -> ()
            n194 = local write "Scans"(w364) -> ()
            n195 = property on="Scan Type" class="Ring (strict)"("Value (Signaling)"=w350) -> ()  [unwired: 2 in, 2 out]
            n196 = case shown="False" w341 {
              selector: w341 -> [_ w390]
              tunnel: w362 -> [w371 w386]
              tunnel: w360 -> [w372 w387]
              tunnel: w361 -> [w369 w389]
              tunnel: [w369 w393] -> w342
              tunnel: [w372 w392] -> w363
              tunnel: [w371 w391] -> w343
              tunnel: [w368 w385] -> w358
              tunnel: w347 -> [w370 _]
              tunnel: w346 -> [w367 _]
              tunnel: w345 -> [w366 _]
              tunnel: w344 -> [_ w384]
              frame False {
                n197 = case shown="1, 4" w370 {
                  tunnel: w369 -> [w376 w379 w382]
                  tunnel: [w373 w378 w381] -> w368
                  tunnel: w367 -> [w375 _ _]
                  tunnel: w366 -> [w374 _ _]
                  frame Default {
                    n198 = Multiply(x=w376, y=w375) -> (x*y=w377:dbl)
                    n199 = Add(x=w377, y=w374) -> (x+y=w373:dbl)
                  }
                  frame 1, 4 {
                    n200 = global read "_Global Configuration.vi" "Calibration"() -> (w380:dbl[][])
                    n201 = call "_Convert Mass to DAC.vi"("Calibration Table"=w380, "Mass"=w379) -> ("DAC Value"=w378:dbl)  [unwired: 2 in, 3 out]
                  }
                  frame 2, 5 {
                    n202 = global read "_Global Configuration.vi" "Calibration 2"() -> (w383:dbl[][])
                    n203 = call "_Convert Mass to DAC.vi"("Calibration Table"=w383, "Mass"=w382) -> ("DAC Value"=w381:dbl)  [unwired: 2 in, 3 out]
                  }
                }
              }
              frame True {
                # "Convert to DAC units"
                n204 = Bundle(w390, "Value 1"=w389, "Value 2"=w387, "Step Size"=w386) -> (w388:T23)  [unwired: 1 out]
                n205 = call "_Switch Lens Property Unit.vi"("Lens Property In"=w388, "Configuration"=w384) -> ("DAC Value"=w385:i32, "Step Size"=w391:dbl, "Count2"=w392:dbl, "Count1"=w393:dbl)  [unwired: 1 in, 1 out]
              }
            }
            n206 = local write "DAC Value"(w358) -> ()
            n207 = local write "Count1"(w342) -> ()
            n208 = local write "Count2"(w363) -> ()
            n209 = local write "Step Size"(w343) -> ()
          }
          event "Scan Type": Value Change {
            n210 = event-data() -> ("NewVal"=w406:u8)  [unwired: 6 out]
            n211 = case shown="1" w406 {
              tunnel: ["Lens Value" "Low Value" "Start Value"] -> w405
              tunnel: ["High Value" "High Value" "Stop Value"] -> w404
              tunnel: ["Low Dwell (ms)" "Low Time (ms)" "Dwell Time (ms)"] -> w403
              tunnel: ["High Dwell (ms)" "High Time (ms)" "Pause Time (ms)"] -> w402
              tunnel: [w411 w416 w418] -> w401
              tunnel: [w411 w416 w418] -> w400
              tunnel: [w411 w416 w418] -> w399
              tunnel: [w411 w416 w418] -> w398
              tunnel: [w411 FALSE w418] -> w397
              frame 0, Default {
                w411 = FALSE
                # "For Single"
              }
              frame 1 {
                w416 = TRUE
                # "For Dual"
              }
              frame 2 {
                w418 = TRUE
                # "For Ramp"
              }
            }
            n212 = property on="Count2" class="DigNum (strict)"("Visible"=w401) -> ()  [unwired: 2 in, 2 out]
            n213 = property on="Time1" class="DigNum (strict)"("Visible"=w400) -> ()  [unwired: 2 in, 2 out]
            n214 = property on="Time2" class="DigNum (strict)"("Visible"=w399) -> ()  [unwired: 2 in, 2 out]
            n215 = property on="Scans" class="DigNum (strict)"("Visible"=w398) -> ()  [unwired: 2 in, 2 out]
            n216 = property on="Step Size" class="DigNum (strict)"("Visible"=w397) -> ()  [unwired: 2 in, 2 out]
            n217 = property on="Count1" class="DigNum (strict)"("Caption.Text"=w405) -> ()  [unwired: 2 in, 2 out]
            n218 = property on="Count2" class="DigNum (strict)"("Caption.Text"=w404) -> ()  [unwired: 2 in, 2 out]
            n219 = property on="Time1" class="DigNum (strict)"("Caption.Text"=w403) -> ()  [unwired: 2 in, 2 out]
            n220 = property on="Time2" class="DigNum (strict)"("Caption.Text"=w402) -> ()  [unwired: 2 in, 2 out]
            n221 = Bundle By Name(cluster=w396, "Update"=TRUE) -> (w395:T17)
          }
          event "Run": Value Change {
            n222 = event-data() -> ()  [unwired: 7 out]
            n223 = stacked-sequence {
              tunnel: w428 -> [_ _ _ w452 _ _]
              tunnel: w427 -> [w432 _ _ _ _ _]
              tunnel: w426 -> [_ _ w437 _ _ _]
              tunnel: [_ _ w436 _ _ _] -> w424
              frame #0 {
                w430 = u8 1 ("Disabled")
                n224 = Flush Queue(queue=w432) -> ()  [unwired: 1 in, 3 out]
                n225 = call <vilib>:"Set Busy.vi"() -> ()  [unwired: 4 in, 8 out]
                n226 = property on="Scan#" class="DigNum (strict)"("Disabled"=w430) -> ()  [unwired: 2 in, 2 out]
                n227 = property on="Acquire" class="Bool (strict)"("Disabled"=w430) -> ()  [unwired: 2 in, 2 out]
                n228 = property on="MCA" class="Bool (strict)"("Disabled"=w430) -> ()  [unwired: 2 in, 2 out]
                n229 = property on="Run" class="Bool"("Visible"=FALSE) -> ()  [unwired: 2 in, 2 out]
                n230 = property on="Cancel" class="Bool"("Visible"=TRUE) -> ()  [unwired: 2 in, 2 out]
              }
              frame #1 {
                n231 = Wait (ms)(milliseconds to wait=u32 180) -> ()  [unwired: 1 out]
              }
              frame #2 {
                w434 = T24 0 items=["Diagnostics", "Tune", "Acquisition"] ("RunModule")
                n232 = case shown="True" "Acquire" {
                  tunnel: w437 -> [w439 w444]
                  tunnel: [w439 w441] -> w436
                  frame False {
                  }
                  frame True {
                    n233 = local read "Data File:"() -> (w445:path)
                    n234 = call "_Get File.vi"("Start Path"=w445) -> ("Seleted File"=w446:path, "Succeeded"=w442:bool)  [unwired: 5 in, 2 out]
                    n235 = local write "Acquire"(w442) -> ()
                    n236 = case shown="True" w442 {
                      tunnel: w446 -> [_ w448]
                      tunnel: w445 -> [w447 _]
                      tunnel: [w447 w448] -> w443
                      frame False {
                      }
                      frame True {
                        n237 = local write "Data File:"(w448) -> ()
                      }
                    }
                    n238 = Bundle By Name(cluster=w444, "Method.Data Path"=w443, "Method.Acquire"=w442) -> (w441:T17)
                    n239 = Unbundle By Name(w441) -> ("Method"=w440:T2)
                    n240 = local write "Method"(w440) -> ()
                  }
                }
                n241 = global write "_Global Configuration.vi" "Run"(TRUE ("Update")) -> ()
                n242 = global write "_Global Configuration.vi" "RunModule"(w434) -> ()
              }
              frame #3 {
                n243 = local read "Scan Type"() -> (w451:u8)
                n244 = Equal?(x=w451, y=u16 1) -> (x = y?=w449:bool)
                n245 = case shown="True" w449 {
                  selector: w449 -> [_ w457]
                  tunnel: w452 -> [w455 _]
                  frame False {
                    w454 = FALSE ("Wait until done")
                    n246 = invoke class="VI" method="Run VI"(reference=w455, "Wait until done"=w454, "Auto Dispose Ref"=w454) -> ()  [unwired: 2 in, 5 out]
                    n247 = local write "Scan#"(u32 0 ("Scan#")) -> ()
                  }
                  frame True {
                    n248 = local write "Dual Run"(w457) -> ()
                    n249 = property on="Dual Run" class="Bool (strict)"("Visible"=w457) -> ()  [unwired: 2 in, 2 out]
                    n250 = call "_Remote Run Dual.vi"() -> ("error out"=w456:errorcluster)  [unwired: 2 in, 5 out]
                    n251 = call "_Handle Error.vi"("error in (no error)"=w456) -> ()  [unwired: 2 in, 5 out]
                  }
                }
              }
              frame #4 {
                n252 = Wait (ms)(milliseconds to wait=u32 800) -> ()  [unwired: 1 out]
              }
              frame #5 {
                n253 = call <vilib>:"Unset Busy.vi"() -> ()  [unwired: 2 in, 10 out]
              }
            }
            n254 = Bundle By Name(cluster=w424, "Running"=TRUE) -> (w423:T17)
          }
          event "Cancel": Value Change {
            n255 = event-data() -> ()  [unwired: 7 out]
            n256 = stacked-sequence {
              tunnel: w461 -> [_ w465 _]
              tunnel: [_ w464 _] -> w460
              tunnel: w459 -> [_ w463 _]
              frame #0 {
                n257 = call <vilib>:"Set Busy.vi"() -> ()  [unwired: 4 in, 8 out]
                n258 = global write "_Global Configuration.vi" "Run"(FALSE ("Update")) -> ()
              }
              frame #1 {
                n259 = local read "Dual Run"() -> (w466:bool)
                n260 = case shown="True" w466 {
                  tunnel: w465 -> [w468 w478]
                  tunnel: [w468 w477] -> w464
                  tunnel: w463 -> [w467 _]
                  frame False {
                    n261 = while {
                      tunnel: w467 -> [w473]
                      stop <- w470 stop-if-true
                      n262 = property class="VI"(reference=w473) -> ("Exec.State"=w472:T15)  [unwired: 1 in, 2 out]
                      n263 = Wait (ms)(milliseconds to wait=u32 180) -> ()  [unwired: 1 out]
                      n264 = Equal?(x=w472, y=T15."Idle") -> (x = y?=w470:bool)
                    }
                  }
                  frame True {
                    w479 = u8 0 ("Disabled")
                    w476 = FALSE
                    n265 = property on="Run" class="Bool"("Visible"=TRUE) -> ()  [unwired: 2 in, 2 out]
                    n266 = property on="Cancel" class="Bool"("Visible"=FALSE) -> ()  [unwired: 2 in, 2 out]
                    n267 = local write "Dual Run"(w476) -> ()
                    n268 = property on="Dual Run" class="Bool (strict)"("Visible"=w476) -> ()  [unwired: 2 in, 2 out]
                    n269 = property on="Acquire" class="Bool (strict)"("Disabled"=w479) -> ()  [unwired: 2 in, 2 out]
                    n270 = property on="MCA" class="Bool (strict)"("Disabled"=w479) -> ()  [unwired: 2 in, 2 out]
                    n271 = property on="Scan#" class="DigNum (strict)"("Disabled"=w479) -> ()  [unwired: 2 in, 2 out]
                    n272 = Bundle By Name(cluster=w478, "Running"=w476) -> (w477:T17)
                    n273 = call "_Remote Communicate.vi"("Command"=_RT_Command."Stop") -> ()  [unwired: 5 in, 4 out]
                  }
                }
              }
              frame #2 {
                n274 = call "_Remote Wait Until Done.vi"() -> ("error out"=w481:errorcluster)  [unwired: 2 in, 1 out]
                n275 = call <vilib>:"Unset Busy.vi"() -> ()  [unwired: 2 in, 10 out]
                n276 = call "_Remote Park Lens.vi"("error in"=w481) -> ()  [unwired: 1 in, 6 out]
              }
            }
          }
          event "BloUpdate": Value Change {
            n277 = event-data() -> ()  [unwired: 7 out]
            n278 = Unbundle By Name(w483) -> ("Running"=w482:bool)
            n279 = local write "BloUpdate"(FALSE) -> ()
            n280 = stacked-sequence {
              seq-local: [_ w487 _ _] -> [_ _ _ w488]
              tunnel: w482 -> [_ w486 _ _]
              frame #0 {
                n281 = call <vilib>:"Set Busy.vi"() -> ()  [unwired: 4 in, 8 out]
              }
              frame #1 {
                n282 = call "_Remote BlockUpdate.vi"("Filter (T)"=FALSE, "Running"=w486) -> ("error out"=w487:errorcluster)  [unwired: 1 in, 4 out]
              }
              frame #2 {
                n283 = call <vilib>:"Unset Busy.vi"() -> ()  [unwired: 2 in, 10 out]
              }
              frame #3 {
                n284 = call "_Handle Error.vi"("error in (no error)"=w488) -> ()  [unwired: 2 in, 5 out]
              }
            }
          }
          event "NewMethod": Value Change {
            n285 = event-data() -> ()  [unwired: 2 out]
            n286 = local write "NewMethod"(FALSE) -> ()
            n287 = Unbundle By Name(w496) -> ("Running"=w490:bool, "Method"=w498:T2)
            n288 = property on="Lens Table" class="MCListbox (strict)"("Value (Signaling)"=0) -> ()  [unwired: 2 in, 2 out]
            n289 = Unbundle By Name(w498) -> ("Q3DC EN"=w493:bool, "Run Mode"=w492:T1, "Acquire"=w509:bool, "MCA"=w508:bool, "Q1DC EN"=w512:bool, "Q1 POL"=w511:bool, "Q3 POL"=w510:bool, "Averaging"=w504:bool, "Log Scale"=w505:bool, "CPS"=w506:bool, "Data Path"=w507:path, "Lenses"=w500:T3[])  [unwired: 1 out]
            n290 = Array Size(array=w500) -> (size(s)=w502:i32)
            n291 = Array Size(array=w499) -> (size(s)=w503:i32)
            n292 = Not Equal?(x=w502, y=w503) -> (x != y?=w501:bool)
            n293 = case shown="True" w501 {
              tunnel: w499 -> [_ w517]
              tunnel: [w514 w515] -> w497
              tunnel: w500 -> [w514 _]
              frame False {
              }
              frame True {
                n294 = for {
                  tunnel: w517 -> [w520] mode=indexing
                  tunnel: T3 {"Scan Type"=0, "Scans"=1, "Time 1"=1.0, "Time 2"=1.0, "Value 1"=0.0, "Value 2"=0.0, "Step Size"=1.0} ("Lenses") -> [w521]
                  tunnel: [w518] -> w515 mode=indexing
                  n295 = Unbundle By Name(w520) -> ("Def+"=w519:dbl)
                  n296 = Bundle By Name(cluster=w521, "Value 1"=w519, "Value 2"=w519) -> (w518:T3)
                }
              }
            }
            n297 = stacked-sequence {
              tunnel: w512 -> [w526 _ _]
              tunnel: w511 -> [w524 _ _]
              tunnel: w510 -> [w525 _ _]
              tunnel: w509 -> [_ _ w546]
              tunnel: w508 -> [_ _ w545]
              tunnel: w507 -> [_ w540 _]
              tunnel: w506 -> [_ w539 _]
              tunnel: w505 -> [_ w538 _]
              tunnel: w504 -> [_ w537 _]
              tunnel: w493 -> [w527 _ _]
              tunnel: w492 -> [_ _ w544]
              tunnel: w490 -> [w522 _ _]
              frame #0 {
                n298 = local write "Q2DC EN"(w527) -> ()
                n299 = local write "Q1DC EN"(w526) -> ()
                n300 = local write "Q1 POL"(w524) -> ()
                n301 = local write "Q2 POL"(w525) -> ()
                n302 = Number To Boolean Array(number=u16 0) -> (Boolean array=w533:bool[])
                n303 = Replace Array Subset(array=w533, new element #1=w524, index #1=0 ("index"), new element #2=w525, index #2=1 ("index"), new element #3=w526, index #3=2 ("index"), new element #4=w527, index #4=3 ("index")) -> (w528:bool[])
                n304 = Boolean Array To Number(Boolean array=w528) -> (number=w523:u16)
                n305 = case shown="False" w522 {
                  tunnel: w523 -> [w535 _]
                  frame False {
                    n306 = call "_Remote Communicate.vi"("DC Param"=w535, "Command"=_RT_Command."Set Pol and DC") -> ()  [unwired: 4 in, 4 out]
                  }
                  frame True {
                  }
                }
              }
              frame #1 {
                n307 = local write "Averaging"(w537) -> ()
                n308 = local write "Log Scale"(w538) -> ()
                n309 = local write "CPS"(w539) -> ()
                n310 = call "_Read Spectrum File.vi"("advisory dialog? (display:T)"=FALSE, "start path  (Not A Path)"=w540) -> ("new file path"=→"Data File:":path, "Scan# out"=w541:u32)  [unwired: 1 in, 5 out]
                n311 = local write "Scan#"(w541) -> ()
              }
              frame #2 {
                n312 = local write "Acquire"(w546) -> ()
                n313 = local write "MCA"(w545) -> ()
                n314 = global read "_Global Configuration.vi" "Spectrum"() -> (w547:i32[])
                n315 = property on="Run Mode" class="Enum (strict)"("Val(Sgnl)"=w544) -> ()  [unwired: 2 in, 2 out]
                n316 = call "_Update Display Property 2.vi"("Spectrum in"=w547) -> ()  [unwired: 7 out]
              }
            }
            n317 = Bundle By Name(cluster=w496, "Method.Negative"=FALSE, "Method.Mass Ranges"=T4[] [], "Method.Lenses"=w497) -> (w495:T17)
          }
          event "Swtich Polarity": Value Change {
            n318 = event-data() -> ()  [unwired: 7 out]
            n319 = Unbundle By Name(w550) -> ("Method.Lenses"=w548:T3[], "Running"=w549:bool)
            n320 = case shown="False" w549 {
              tunnel: w550 -> [w557 w563]
              tunnel: [w555 w563] -> w551
              tunnel: w548 -> [w553 _]
              frame False {
                n321 = local read "Lens Table"() -> (w558:i32)
                n322 = local read "Count1"() -> (w562:dbl)
                n323 = local read "Count2"() -> (w561:dbl)
                n324 = call "_Switch Polarity.vi"("Lenses"=w553, "Start Value"=w562, "Stop Value"=w561, "index"=w558, "Unit"="Unit") -> ("Lenses 2"=w556:T3[], "Start Value 2"=w560:dbl, "Stop Value 2"=w559:dbl)  [unwired: 1 in]
                n325 = local write "Count1"(w560) -> ()
                n326 = local write "Count2"(w559) -> ()
                n327 = Bundle By Name(cluster=w557, "Method.Lenses"=w556, "Update"=TRUE) -> (w555:T17)
              }
              frame True {
                n328 = One Button Dialog(message="You must wait until the run is finish before you can switch lens polarity.") -> ()  [unwired: 2 out]
              }
            }
          }
          event "Q1DC EN", "Q1 POL", "Q2 POL", "Q2DC EN": Value Change {
            n329 = event-data() -> ()  [unwired: 2 out]
            n330 = Number To Boolean Array(number=u16 0) -> (Boolean array=w577:bool[])
            n331 = Replace Array Subset(array=w577, new element #1="Q1 POL", index #1=0 ("index"), new element #2="Q2 POL", index #2=1 ("index"), new element #3="Q1DC EN", index #3=2 ("index"), new element #4="Q2DC EN", index #4=3 ("index")) -> (w568:bool[])
            n332 = Unbundle By Name(w566) -> ("Running"=w565:bool)
            n333 = Bundle By Name(cluster=w566, "Method.Q1DC EN"="Q1DC EN", "Method.Q1 POL"="Q1 POL", "Method.Q3 POL"="Q2 POL", "Method.Q3DC EN"="Q2DC EN") -> (w579:T17)
            n334 = Boolean Array To Number(Boolean array=w568) -> (number=w567:u16)
            n335 = case shown="False" w565 {
              tunnel: w567 -> [w582 _]
              frame False {
                n336 = call "_Remote Communicate.vi"("DC Param"=w582, "Command"=_RT_Command."Set Pol and DC") -> ("error out"=w583:errorcluster)  [unwired: 4 in, 3 out]
                n337 = property on="BloUpdate" class="Bool (strict)"("Value (Signaling)"=TRUE) -> ()  [unwired: 2 in, 2 out]
                n338 = call "_Handle Error.vi"("error in (no error)"=w583) -> ()  [unwired: 2 in, 5 out]
              }
              frame True {
              }
            }
            n339 = Unbundle By Name(w579) -> ("Method"=w580:T2)
            n340 = local write "Method"(w580) -> ()
          }
          event "CPS", "Averaging", "Log Scale": Value Change {
            n341 = event-data() -> ()  [unwired: 7 out]
            n342 = stacked-sequence {
              tunnel: w586 -> [w592 w594]
              tunnel: [w588 _] -> w585
              frame #0 {
                n343 = Bundle By Name(cluster=w592, "Method.Averaging"="Averaging", "Method.Log Scale"="Log Scale", "Method.CPS"="CPS") -> (w588:T17)
                n344 = Unbundle By Name(w588) -> ("Method"=w587:T2)
                n345 = local write "Method"(w587) -> ()
              }
              frame #1 {
                n346 = Unbundle By Name(w594) -> ("Running"=w593:bool)
                n347 = case shown="False" w593 {
                  frame False {
                    n348 = global read "_Global Configuration.vi" "Spectrum"() -> (w595:i32[])
                    n349 = call "_Update Display Property 2.vi"("Spectrum in"=w595) -> ()  [unwired: 7 out]
                  }
                  frame True {
                  }
                }
              }
            }
          }
          event "Acquire", "MCA": Value Change {
            n350 = event-data() -> ()  [unwired: 7 out]
            n351 = local read "Acquire"() -> (w599:bool)
            n352 = Bundle By Name(cluster=w600, "Method.Acquire"=w599, "Method.MCA"="MCA") -> (w596:T17)
            n353 = Unbundle By Name(w596) -> ("Method"=w597:T2)
            n354 = local write "Method"(w597) -> ()
          }
          event "Scan#": Value Change {
            n355 = event-data() -> ("NewVal"=w605:u32)  [unwired: 1 out]
            n356 = Unbundle By Name(w602) -> ("Running"=w601:bool)
            n357 = global read "_Global Configuration.vi" "# of Scans"() -> (w604:i32)
            n358 = In Range and Coerce(upper limit=w604, x=w605, lower limit=u32 1) -> (coerced(x)=w603:u32)  [unwired: 1 out]
            n359 = case shown="False" w601 {
              tunnel: w603 -> [w609 _]
              frame False {
                n360 = local read "Data File:"() -> (w611:path)
                n361 = call "_Read Spectrum File.vi"("advisory dialog? (display:T)"=FALSE, "Scan#"=w609, "start path  (Not A Path)"=w611) -> ("error"=w613:bool, "TIC"=w612:u32, "error out"=w607:errorcluster, "Scan# out"=w610:u32)  [unwired: 3 out]
                n362 = case shown="False" w613 {
                  tunnel: w612 -> [_ _]
                  tunnel: w610 -> [w615 _]
                  tunnel: w607 -> [_ w616]
                  frame False {
                    n363 = global read "_Global Configuration.vi" "Spectrum"() -> (w614:i32[])
                    n364 = local write "Scan#"(w615) -> ()
                    n365 = call "_Update Display Property 2.vi"("Spectrum in"=w614) -> ()  [unwired: 7 out]
                  }
                  frame True {
                    n366 = call "_Handle Error.vi"("error in (no error)"=w616) -> ()  [unwired: 2 in, 5 out]
                  }
                }
              }
              frame True {
                n367 = One Button Dialog(message="You must wait until the run is finish before you can load another spectrum.") -> ()  [unwired: 2 out]
              }
            }
          }
          event "Count1", "Count2", "Time1", "Time2", "Scans", "Step Size": Value Change {
            n368 = event-data() -> ()  [unwired: 2 out]
            n369 = Bundle By Name(cluster=w619, "Update"=TRUE) -> (w618:T17)
          }
          event "Unit": Value Change {
            n370 = event-data() -> ("NewVal"=w621:bool)  [unwired: 1 out]
            n371 = local read "Lens Table"() -> (w626:i32)
            n372 = local read "Step Size"() -> (w634:dbl)
            n373 = local read "Count1"() -> (w633:dbl)
            n374 = local read "Count2"() -> (w632:dbl)
            n375 = Index Array(array=w627, index=w626) -> (element=w625:T9)
            n376 = Bundle("NewVal"=w621, "Count1"=w633, "Count2"=w632, "Step Size"=w634) -> (w631:T25)  [unwired: 1 out]
            n377 = call "_Switch Lens Property Unit.vi"("Lens Property In"=w631, "Configuration"=w625) -> ("Step Size"=w628:dbl, "Count2"=w629:dbl, "Count1"=w630:dbl)  [unwired: 1 in, 2 out]
            n378 = local write "Count1"(w630) -> ()
            n379 = local write "Count2"(w629) -> ()
            n380 = local write "Step Size"(w628) -> ()
            n381 = Bundle By Name(cluster=w623, "Method.Unit"=w621, "Update"=TRUE) -> (w622:T17)
          }
          event Value Change {
            n382 = event-data() -> ("NewVal"=w636:T1)  [unwired: 1 out]
            n383 = Bundle By Name(cluster=w637, "Method.Run Mode"=w636) -> (w635:T17)
          }
        }
      }
    }
    frame #2 {
      n384 = property class="VI"(reference=w642, error in=w641, "Front Panel Window:Open"=TRUE) -> (reference out=w643:refnum<vi>, error out=w644:errorcluster)
      n385 = Close Reference(reference=w643, error in (no error)=w644) -> (error out=w640:errorcluster)
      n386 = Close Reference(reference=w646, error in (no error)=w640) -> (error out=w639:errorcluster)
      n387 = Release Queue(queue=w647, error in (no error)=w639) -> (error out=w638:errorcluster)  [unwired: 3 out]
    }
  }
  n388 = Merge Errors(w3, w1, w2) -> (→"Error Out":errorcluster)
